vi "FG RBT Services.vi"(1 "FG Action (Read)":T2, 2 "Services in":T1[](array[typedef])) -> (0 "Services out":T1[](array[typedef]))   [LabVIEW 2011]
uses:
  cRIO/Functional Global Variables/Actions for FG's.ctl
  Support Files/ServiceRec.ctl
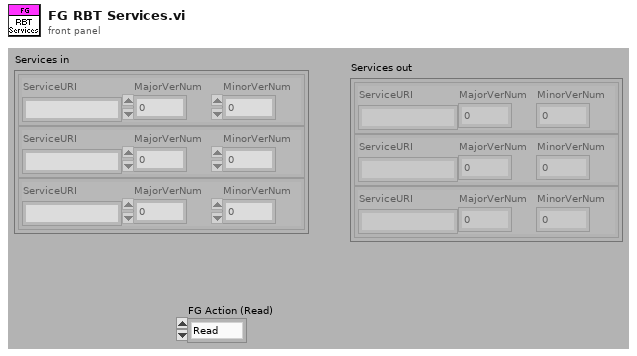
[diagram p1: front panel]
types:
  T1 = typedef "ServiceRec.ctl" = cluster{"ServiceURI":string, "MajorVerNum":u8, "MinorVerNum":u8}
  T2 = typedef "Actions for FG's.ctl" = enum16{"Read", "Write"}
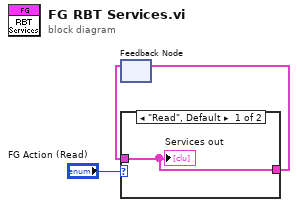
[diagram p0: block diagram]
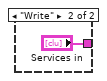
[diagram p2: hidden frame]
diagram:
  n1 = feedback #1() -> (w1:T1[])  [unwired: 1 in]
  n2 = case shown="\"Read\", Default" "FG Action (Read)" {
    tunnel: w1 -> [w4 _]
    tunnel: [w4 "Services in"] -> w2
    frame "Read", Default {
      "Services out" <- w4
    }
    frame "Write" {
    }
  }
  n3 = feedback-in #1(w2) -> ()
